vi "FPGA Read By Name - I64.vi"(8 "error in (no error)":errorcluster, 10 "Indicator":string, 11 "FPGA Session In":refnum<class "FPGA Interface Base.lvclass">) -> (0 "error out":errorcluster, 2 "Value":i64, 3 "FPGA Session Out":refnum<class "FPGA Interface Base.lvclass">)   [LabVIEW 2010, in "FPGA Interface Base.lvclass"]
doc: "Reads a signed 64-bit integer value from a given indicator or control."
uses:
  <userlib>/_FPGA Interface Advanced Tools/FPGA Interface Base/FPGA Interface Base.lvclass
  <vilib>/rvi/DataTransferAndStorage/Container/Common/niFpgaDataTypeControl.ctl
  <userlib>/_FPGA Interface Advanced Tools/FPGA Interface Base/FPGA Interface Base.lvclass/FPGA Interface Base.ctl
  <vilib>/Utility/error.llb/Error Cluster From Error Code.vi
  <userlib>/_FPGA Interface Advanced Tools/FPGA Interface Base/Accessors/FPGA Read Session.vi
  <userlib>/_FPGA Interface Advanced Tools/FPGA Interface Wrapper/FPGA Interface Wrapper.lvlib
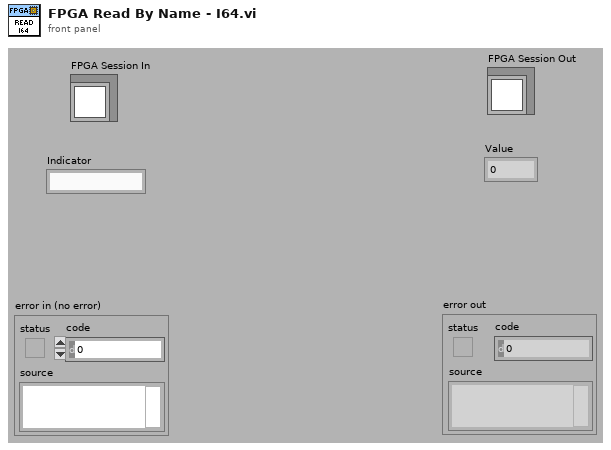
[diagram p1: front panel]
types:
  T1 = typedef "niFpgaDataTypeControl.ctl" = enum32{"Boolean", "I8", "I16", "I32", "I64", "U8", "U16", "U32", "U64", "FXP", "CustomControl"}
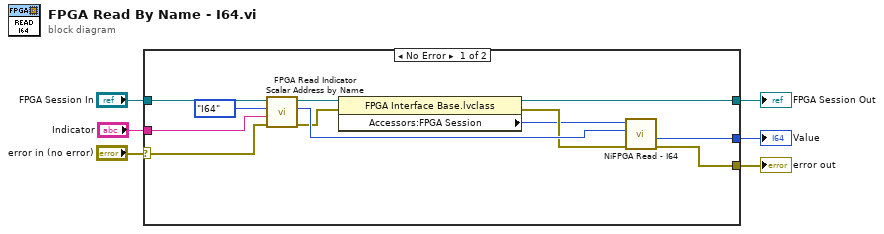
[diagram p0: block diagram]
diagram:
  n1 = case shown="No Error" "error in (no error)" {
    selector: "error in (no error)" -> [w9 w20]
    tunnel: [w7 w20] -> w1
    tunnel: [w8 w19] -> w3
    tunnel: [w18 _] -> w2
    tunnel: "FPGA Session In" -> [w10 w19]
    tunnel: "Indicator" -> [w16 _]
    frame No Error {
      n2 = call <userlib>:"FPGA Read Indicator Scalar Address by Name.vi"("error in (no error)"=w9, "Name"=w16, "Data Type"=niFpgaDataTypeControl."I64", "FPGA Interface Base in"=w10) -> ("error out"=w14:errorcluster, "Address"=w15:u32, "FPGA Interface Base out"=w13:refnum<class "FPGA Interface Base.lvclass">)  [unwired: 4 in, 1 out]
      n3 = property class="FPGA Interface Base.lvclass"(reference=w13, error in=w14) -> (reference out=w8:refnum<class "FPGA Interface Base.lvclass">, error out=w12:errorcluster, "Accessors:FPGA Session"=w11:u32)
      n4 = call <userlib>:"NiFPGA Read - I64.vi"("error in (no error)"=w12, "Indicator"=w15, "Session"=w11) -> ("error out"=w7:errorcluster, "Value"=w18:i64)  [unwired: 6 in, 1 out]
    }
    frame Error {
    }
  }
  "error out" <- w1
  "FPGA Session Out" <- w3
  "Value" <- w2
